vi "propdotnet.vi"   [LabVIEW 2014]
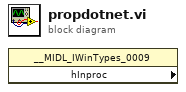
[diagram p0: block diagram]
diagram:
  n1 = property class="__MIDL_IWinTypes_0009" props=["hInproc"]() -> ()  [unwired: 2 in, 3 out]
